vi "Get Localized Phrase.vi"(8 "error in":errorcluster, 9 "Target Language (current lang)":string, 10 "Key":string) -> (0 "error out":errorcluster, 2 "Translated Phrase":string)   [LabVIEW 2017, in "JKI Simple Localization.lvlib"]
doc: "Gets the localized phrase by key from the current dictionary.\n\nKey: Unique identifier defined in the dictionary\nTarget Language (current lang): Optional input. Set this to translate a phase to a language other than the current language."
uses:
  JKI Simple Localization.lvlib
  Definitions/Private/Localization FGV Action -- Enum.ctl
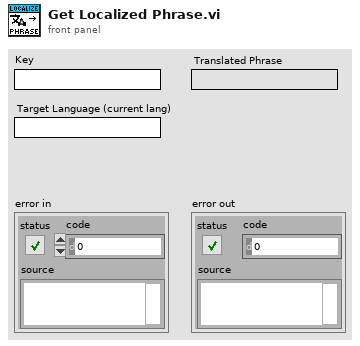
[diagram p1: front panel]
types:
  T1 = typedef "JKI Simple Localization.lvlib/Localization FGV Action -- Enum.ctl" = enum16{"Read Dictionary", "Translate VIs", "Register VI", "Get Languages", "Translate Phrase", "Translate VI", "Unregister"}
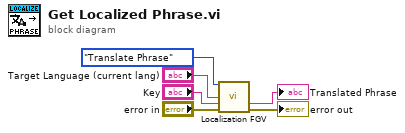
[diagram p0: block diagram]
diagram:
  n1 = call "Localization FGV.vi"("Action"=Localization_FGV_Action_--_Enum."Translate Phrase", "Target Language"="Target Language (current lang)", "UID"="Key", "error in"="error in") -> ("Translated Word"=→"Translated Phrase":string, "error out"=→"error out":errorcluster)  [unwired: 7 in, 3 out]
